vi "SS2 Live_Save Data to HDF5.vi"(6 "Compression":bool, 8 "error in (no error)":errorcluster, 9 "SS2 Live Gate Data Q Name":string="SS2 Live Gate Data Q", 10 "10-bit Gate Image":bool, 11 "HDF5 ref":T1 format="%.0x") -> (0 "error out":errorcluster)   [LabVIEW 2019]
uses:
  <vilib>/addons/h5labview2/base/hid_t.ctl
  <vilib>/addons/h5labview2/file/H5F.lvlib
  <vilib>/addons/h5labview2/group/H5G.lvlib
  Notebook/Notebook.lvlib
  Rich Text Box/Rich Text Box.lvlib
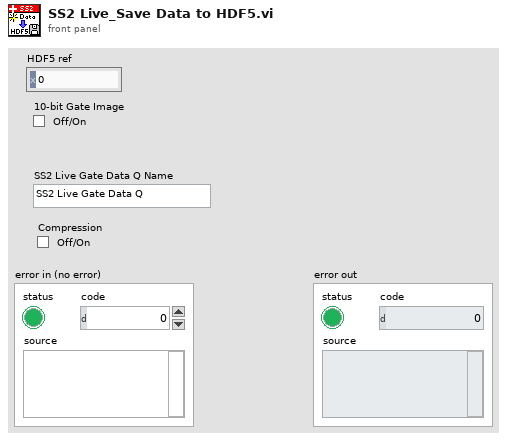
[diagram p1: front panel]
types:
  T1 = typedef "hid_t.ctl" = i32
  T2 = typedef "SS2 Live_File Saving Task Information.ctl" = cluster{"File Path":string, "# Saved Images":i32, "# Images (Total)":i32, "File Size (Bytes)":i64}
  T3 = typedef "Rich Text Box.lvlib/Text Formatting.ctl" = cluster{"Font":string, "Text Color":T4, "Text Background Color":T4, "Text Style":enum16{"Regular", "Bold", "Italic", "Underline", "Strikeout"}, "Font Size (Points)":dbl, "Text Alignment":i32}
  T4 = typedef "Rich Text Box.lvlib/Text Colors.ctl" = enum16{"Unchanged", "Black", "Blue", "Gray", "Green", "Red", "White"}
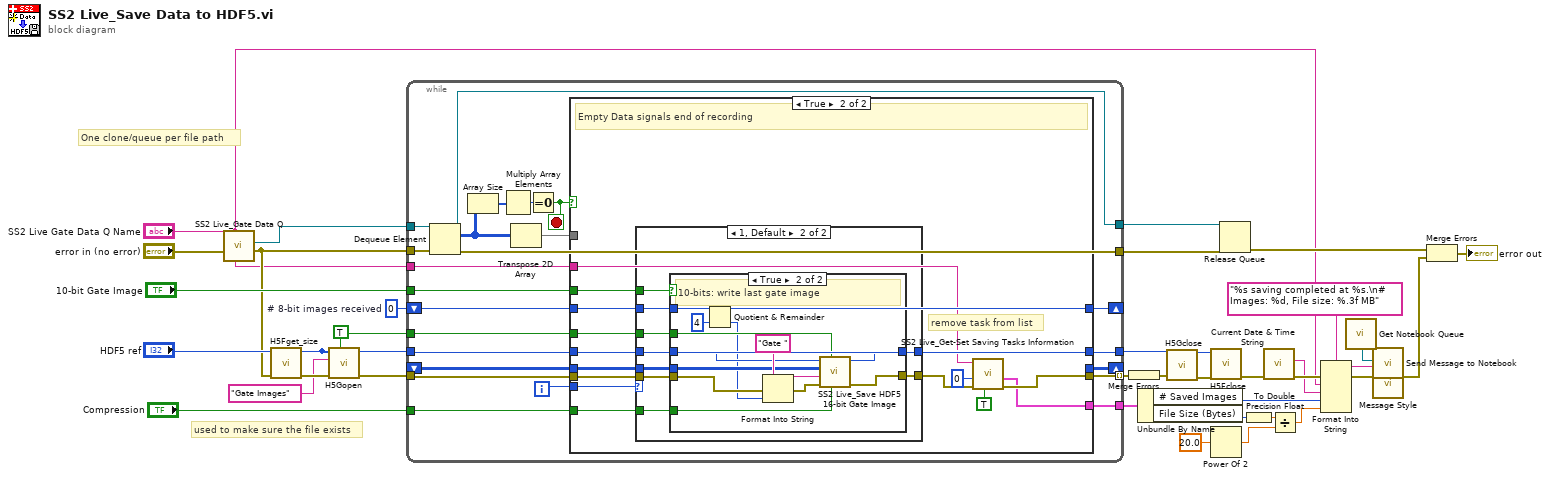
[diagram p0: block diagram]
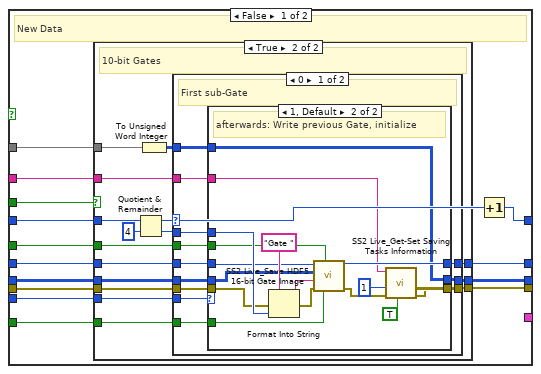
[diagram p2: hidden frame]
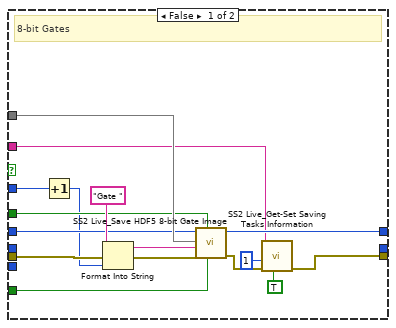
[diagram p3: hidden frame]
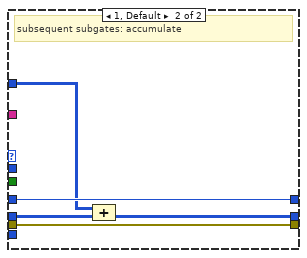
[diagram p5: hidden frame]
diagram:
  w33 = TRUE ("create? (F)")
  w36 = 0  # # 8-bit images received
  # "One clone/queue per file path"
  # "used to make sure the file exists"
  n1 = call "SS2 Live_Gate Data Q.vi"("error in (no error)"="error in (no error)", "SS2 Live Gate Data Q Name"="SS2 Live Gate Data Q Name") -> ("error out"=w19:errorcluster, "SS2 Live Gate Data Q"=w23:refnum<queue>)  [unwired: 4 in]
  n2 = call <vilib>:"H5Fget_size.vi"("error in (no error)"=w19, "ref in"="HDF5 ref") -> ("error out"=w35:errorcluster, "ref out"=w27:T1)  [unwired: 7 in, 1 out]
  n3 = call <vilib>:"H5Gopen.vi"("create? (F)"=w33, "error in (no error)"=w35, "name"="Gate Images", "ref in"=w27) -> ("error out"=w34:errorcluster, "group out"=w31:T1)  [unwired: 6 in]
  n4 = while {
    tunnel: w23 -> [w61]
    tunnel: [w60] -> w38
    tunnel: w31 -> [w59]
    tunnel: w34 -> [w43]
    shift-right: [w51] -> _
    shift-left: w36 -> [w58]
    tunnel: w33 -> [w57]
    tunnel: [w56] -> w30 mode=indexing
    tunnel: [w55] -> w29
    tunnel: "10-bit Gate Image" -> [w49]
    shift-right: [w47] -> _
    shift-left: _ -> [w48]
    tunnel: [w45] -> w25
    tunnel: w19 -> [w42]
    tunnel: "SS2 Live Gate Data Q Name" -> [w41]
    tunnel: [w40] -> w8
    tunnel: "Compression" -> [w39]
    i -> [w46]
    stop <- w52 stop-if-true
    n5 = Dequeue Element(queue=w61, error in (no error)=w42) -> (queue out=w60:refnum<queue>, element=w50:u8[][], error out=w45:errorcluster)  [unwired: 1 in, 1 out]
    n6 = Array Size(array=w50) -> (size(s)=w53:i32[])
    n7 = Multiply Array Elements(1:w53) -> (0:w54:i32)
    n8 = Transpose 2D Array(2D array=w50) -> (transposed array=w44:u8[][])
    n9 = Equal To 0?(x=w54) -> (x = 0?=w52:bool)
    n10 = case shown="True" w52 {
      tunnel: w59 -> [w74 w157]
      tunnel: w43 -> [w71 w155]
      tunnel: w58 -> [w63 w154]
      tunnel: w57 -> [w75 w146]
      tunnel: [w65 w152] -> w56
      tunnel: [w73 w156] -> w55
      tunnel: [w72 w154] -> w51
      tunnel: w44 -> [w69 _]
      tunnel: w49 -> [w70 w147]
      tunnel: w48 -> [w68 w158]
      tunnel: [w67 _] -> w47
      tunnel: w46 -> [w66 w144]
      tunnel: w41 -> [w64 w151]
      tunnel: [_ w149] -> w40
      tunnel: w39 -> [w62 w145]
      frame False {
        # "New Data"
        n11 = case shown="True" w70 {
          tunnel: w75 -> [w83 w104]
          tunnel: [w80 w102] -> w65
          tunnel: w74 -> [w85 w106]
          tunnel: [w84 w105] -> w73
          tunnel: w71 -> [w91 w103]
          tunnel: w63 -> [w89 w93]
          tunnel: w69 -> [w86 w107]
          tunnel: w68 -> [_ w100]
          tunnel: [_ w98] -> w67
          tunnel: w66 -> [_ w101]
          tunnel: w64 -> [w78 w97]
          tunnel: w62 -> [w76 w92]
          frame False {
            # "8-bit Gates"
            n12 = Increment(x=w89) -> (x+1=w82:i32)
            n13 = Format Into String(initial string="Gate ", error in=w91, w82) -> (resulting string=w87:string, error out=w88:errorcluster)  [unwired: 1 in]
            n14 = call "SS2 Live_Save HDF5 8-bit Gate Image.vi"("Compression"=w76, "Replace?"=w83, "error in (no error)"=w88, "Image Name"=w87, "Data"=w86, "ref in"=w85) -> ("error out"=w81:errorcluster, "ref out"=w84:T1)  [unwired: 4 in]
            n15 = call "SS2 Live_Get-Set Saving Tasks Information.vi"("Get (F)/Set"=TRUE, "error in (no error)"=w81, "# New Images Saved (1)"=1 ("# New Images Saved"), "File Path"=w78) -> ("error out"=w80:errorcluster)  [unwired: 4 in, 3 out]
          }
          frame True {
            # "10-bit Gates"
            n16 = Quotient & Remainder(x=w93, y=4) -> (x-y*floor(x/y)=w94:i32, floor(x/y)=w95:i32)
            n17 = To Unsigned Word Integer(number=w107) -> (unsigned 16bit integer=w99:u16[][])
            n18 = case shown="0" w94 {
              tunnel: w106 -> [w119 w142]
              tunnel: [w118 w142] -> w105
              tunnel: w104 -> [w117 _]
              tunnel: w103 -> [w116 w143]
              tunnel: [w115 w143] -> w102
              tunnel: w101 -> [w114 _]
              tunnel: w95 -> [w113 _]
              tunnel: w100 -> [w111 w141]
              tunnel: w99 -> [w112 w140]
              tunnel: [w110 w139] -> w98
              tunnel: w97 -> [w109 _]
              tunnel: w92 -> [w108 _]
              frame 0 {
                # "First sub-Gate"
                n19 = case shown="1, Default" w114 {
                  tunnel: w119 -> [w122 w133]
                  tunnel: [w122 w138] -> w118
                  tunnel: w117 -> [_ w132]
                  tunnel: w116 -> [w121 w134]
                  tunnel: [w121 w127] -> w115
                  tunnel: w113 -> [_ w136]
                  tunnel: w112 -> [w120 w129]
                  tunnel: [w120 w129] -> w110
                  tunnel: w111 -> [_ w130]
                  tunnel: w109 -> [_ w125]
                  tunnel: w108 -> [_ w123]
                  frame 0 {
                    # "First Call: initialize"
                  }
                  frame 1, Default {
                    # "afterwards: Write previous Gate, initialize"
                    n20 = Format Into String(initial string="Gate ", error in=w134, w136) -> (resulting string=w131:string, error out=w135:errorcluster)  [unwired: 1 in]
                    n21 = call "SS2 Live_Save HDF5 16-bit Gate Image.vi"("Compression"=w123, "Replace?"=w132, "error in (no error)"=w135, "Image Name"=w131, "Data"=w130, "ref in"=w133) -> ("error out"=w128:errorcluster, "ref out"=w138:T1)  [unwired: 4 in]
                    n22 = call "SS2 Live_Get-Set Saving Tasks Information.vi"("Get (F)/Set"=TRUE, "error in (no error)"=w128, "# New Images Saved (1)"=1, "File Path"=w125) -> ("error out"=w127:errorcluster)  [unwired: 4 in, 3 out]
                  }
                }
              }
              frame 1, Default {
                # "subsequent subgates: accumulate"
                n23 = Compound Arithmetic op=ADD(w140, w141) -> (w139:u16[][])
              }
            }
          }
        }
        n24 = Increment(x=w63) -> (x+1=w72:i32)
      }
      frame True {
        # "remove task from list"
        # "Empty Data signals end of recording"
        n25 = case shown="1, Default" w144 {
          tunnel: w158 -> [_ w169]
          tunnel: w157 -> [w160 w168]
          tunnel: [w160 w167] -> w156
          tunnel: w155 -> [w159 w166]
          tunnel: w154 -> [_ w165]
          tunnel: [w159 w164] -> w153
          tunnel: w147 -> [_ w163]
          tunnel: w146 -> [_ w162]
          tunnel: w145 -> [_ w161]
          frame 0 {
            # "no data ever received (FPGA timeout?)"
          }
          frame 1, Default {
            n26 = case shown="True" w163 {
              tunnel: w169 -> [_ w181]
              tunnel: w168 -> [w171 w180]
              tunnel: [w171 w179] -> w167
              tunnel: w166 -> [w170 w178]
              tunnel: [w170 w177] -> w164
              tunnel: w165 -> [_ w174]
              tunnel: w162 -> [_ w176]
              tunnel: w161 -> [_ w172]
              frame False {
                # "8-bit data: nothing to do"
              }
              frame True {
                # "10-bits: write last gate image"
                n27 = Quotient & Remainder(x=w174, y=4) -> (floor(x/y)=w173:i32)  [unwired: 1 out]
                n28 = Format Into String(initial string="Gate ", error in=w178, w173) -> (resulting string=w182:string, error out=w183:errorcluster)  [unwired: 1 in]
                n29 = call "SS2 Live_Save HDF5 16-bit Gate Image.vi"("Compression"=w172, "Replace?"=w176, "error in (no error)"=w183, "Image Name"=w182, "Data"=w181, "ref in"=w180) -> ("error out"=w177:errorcluster, "ref out"=w179:T1)  [unwired: 4 in]
              }
            }
          }
        }
        n30 = call "SS2 Live_Get-Set Saving Tasks Information.vi"("Get (F)/Set"=TRUE, "error in (no error)"=w153, "# New Images Saved (1)"=0 ("# New Images Saved"), "File Path"=w151) -> ("error out"=w152:errorcluster, "Complete Saving Task Information"=w149:T2)  [unwired: 4 in, 2 out]
      }
    }
  }
  n31 = Merge Errors(w30) -> (w24:errorcluster)
  n32 = Unbundle By Name(w8) -> ("# Saved Images"=w7:i32, "File Size (Bytes)"=w6:i64)
  n33 = call <vilib>:"H5Gclose.vi"("error in (no error)"=w24, "group in"=w29) -> ("error out"=w28:errorcluster)  [unwired: 9 in]
  n34 = call <vilib>:"H5Fclose.vi"("error in (no error)"=w28, "ref"=w27) -> ("error out"=w12:errorcluster)  [unwired: 9 in]
  n35 = Power Of 2(x=20.0) -> (2^x=w4:dbl)
  n36 = Release Queue(queue=w38, error in (no error)=w25) -> (error out=w37:errorcluster)  [unwired: 1 in, 2 out]
  n37 = To Double Precision Float(number=w6) -> (double precision float=w2:dbl)
  n38 = call "Current Date & Time String.vi"("Error In"=w12) -> ("Error Out"=w11:errorcluster, "time string"=w10:string)  [unwired: 8 in, 1 out]
  n39 = Divide(x=w2, y=w4) -> (x/y=w3:dbl)
  n40 = Format Into String(format string="%s saving completed at %s.\n# Images: %d, File size: %.3f MB", error in=w11, "SS2 Live Gate Data Q Name", w10, w7, w3) -> (resulting string=w14:string, error out=w15:errorcluster)  [unwired: 1 in]
  n41 = call "Get Notebook Queue.vi"() -> ("Notebook Queue"=w18:refnum<queue>)  [unwired: 9 in]
  n42 = call "Message Style.vi"() -> ("Message Formatting"=w16:T3)
  n43 = call "Send Message to Notebook.vi"("Notebook Queue"=w18, "Message"=w14, "Error In"=w15, "Text Formatting"=w16) -> ("Error Out"=w17:errorcluster)  [unwired: 15 in]
  n44 = Merge Errors(w37, w17) -> (→"error out":errorcluster)
